vi "Rx_with scope_delta time.vi"() -> ()   [LabVIEW 2021]
uses:
  use with scope/states_for scope.ctl
  <instrlib>/niScope/Controls/niScope trigger source digital.ctl
  use with scope/scope trig type.ctl
  CTL/user config.ctl
  <vilib>/userdefined/High Color/nirio_resource_hc.ctl
  classes/5785_3.2GHz_one channel/5785_3.2GHz_one channel.lvclass
  C:/Users/PXIe8108_Demo/Documents/CHAIM DATA/chaim/5785_sync_for_elbit/tx_pulse/pulse Tx Folder_lv_21/EMEA_ADG_EW_Multi_Emitter_Scenarios/classes/device_type/device_type.lvclass
  classes/5785_2_x_1600MHz/5785_2_x_1600MHz.lvclass
  <instrlib>/niScope/Configure/Trigger/niScope Configure Trigger Edge.vi
  <instrlib>/niScope/Configure/Trigger/niScope Configure Trigger Digital.vi
  <instrlib>/niScope/Acquire/Fetch/niScope Multi Fetch WDT.vi
  <vilib>/Analysis/1siggen.llb/Ramp Pattern by Delta.vi
  classes/device_type/device_type.lvclass
  <vilib>/Analysis/NI_AALBase.lvlib
panel:
  in  "mode":T1(ring)=enum."5785 - 2*180MHz"
  in  "num of nano between channels":dbl
  out "delta range":cluster{dbl[], dbl[]}[](graph)=[{[200000.0, 200000.0, 200000.0, 200000.0, 200000.0, 200000.0, 200000.0, 200000.0, 200000.0, 200000.0, 200000.0, 200000.0, 200000.0, 200000.0, 200000.0, 200000.0, 200000.0, 200000.0, 200000.0, 200000.0, 200000.0, 200000.0, 200000.0, 200000.0, 200000.0, 200000.0, 200000.0, 200000.0, 200000.0, 200000.0, 200000.0, 200000.0, 200000.0, 200000.0, 200000.0, 200000.0, 200000.0, 200000.0, 200000.0, 200000.0, 200000.0, 200000.0, 200000.0, 200000.0, 200000.0, 200000.0, 200000.0, 200000.0, 200000.0, 200000.0, 200000.0, 200000.0, 200000.0, 200000.0, 200000.0, 200000.0, 200000.0, 200000.0, 200000.0, 200000.0, 200000.0, 200000.0, 200000.0, 200000.0, 200000.0, 200000.0, 200000.0, 200000.0, 200000.0, 200000.0, 200000.0, 200000.0, 200000.0, 200000.0, 200000.0, 200000.0, 200000.0, 200000.0, 200000.0, 200000.0, 200000.0, 200000.0, 200000.0, 200000.0, 200000.0, 200000.0, 200000.0, 200000.0, 200000.0, 200000.0, 200000.0, 200000.0, 200000.0, 200000.0, 200000.0, 200000.0, 200000.0, 200000.0, 200000.0, 200000.0, 200000.0, 200000.0, 200000.0, 200000.0, 200000.0, 200000.0, 200000.0, 200000.0, 200000.0, 200000.0, 200000.0, 200000.0, 200000.0, 200000.0, 200000.0, 200000.0, 200000.0, 200000.0, 200000.0, 200000.0, 200000.0, 200000.0, 200000.0, 200000.0, 200000.0, 200000.0, 200000.0, 200000.0, 200000.0, 200000.0, 200000.0, 200000.0, 200000.0, 200000.0, 200000.0, 200000.0, 200000.0, 200000.0, 200000.0, 200000.0, 200000.0, 200000.0, 200000.0, 200000.0, 200000.0, 200000.0, 200000.0, 200000.0, 200000.0, 200000.0, 200000.0, 200000.0, 200000.0, 200000.0, 200000.0, 200000.0, 200000.0, 200000.0, 200000.0, 200000.0, 200000.0, 200000.0], [-1.1815539075178094e-09, -1.1735940937302077e-09, 1.5173838718910703e-08, 1.1955568102002144e-08, 9.78047503704438e-09, 8.264037714514417e-09, 1.529550371572841e-08, 6.153523621009663e-09, 1.1997855926281773e-08, 1.0927362590376289e-08, 9.887324902811088e-09, 9.038956474978476e-09, 8.292742399894633e-09, 1.2053931898903102e-08, 1.538426720065763e-08, 6.832846135215369e-09, 1.3740200297546108e-08, 9.46442253064597e-09, -1.1883506176644005e-09, 2.0508825034904294e-08, 1.5174786625616252e-08, 1.1935071282531135e-08, 9.80493401925778e-09, 8.257336005754769e-09, 7.0956615944276564e-09, 1.3487845511222259e-08, 1.2094480889406986e-08, 1.089261531442171e-08, 9.913567475194577e-09, 1.910663676209515e-08, 1.3123609836224933e-08, 1.1936135569633917e-08, 7.184052554087248e-09, 6.482600684801582e-09, 9.916355201753322e-09, 9.171984461823013e-09, -1.1852903081453406e-09, 2.050388125119498e-08, 1.518068337268196e-08, 1.1954260133113712e-08, 2.0742580365296452e-08, 1.7653907625202556e-08, 1.5293914297246374e-08, 1.3515559364203364e-08, 1.8667553143179976e-08, 1.0837617655762007e-08, 9.826992215344217e-09, 9.018459328566678e-09, 8.301810464903247e-09, 1.2225356932776049e-08, 1.1088317456725054e-08, 1.429163756670896e-08, 6.338322277762927e-09, 5.658937157317996e-09, -1.1859513377188706e-09, -1.1768632264807821e-09, 1.5176432920689697e-08, 1.1960557492042426e-08, 9.826527517207432e-09, 8.233890970330685e-09, 7.106771544471849e-09, 2.0819609779305756e-08, 1.2022157269413583e-08, 1.0826222265674733e-08, 4.390260251308792e-09, 9.068177768285387e-09, 1.7713380407029765e-08, 1.2032988585217391e-08, 1.553451803342905e-08, 6.7977589478599845e-09, 1.3492854561959393e-08, 9.043047258420847e-09, -1.1866718047880568e-09, -1.168161773402244e-09, 1.516217105332762e-08, 1.1939343025384006e-08, 2.0737754271691665e-08, 8.226647777832114e-09, 2.3577958129288165e-08, 1.3539817026490345e-08, 1.2010466453281697e-08, 1.0798456547886599e-08, 9.887342741386966e-09, 9.049870830215513e-09, 1.7723341785010418e-08, 1.2062780513672624e-08, 7.134556607343257e-09, 1.8398769060708582e-08, 1.3532338226772846e-08, 9.478644459473435e-09, -1.1899547685286963e-09, 2.049997443513712e-08, -1.1591381137724966e-09, 2.5083063203259373e-08, 9.758059998776298e-09, 8.208837169304024e-09, 1.5304059904417955e-08, 1.3471675031236374e-08, 1.2010095862450544e-08, 4.8943541112937966e-09, 9.79197639725171e-09, 1.914853386823088e-08, 3.4211602777591907e-09, 1.2148997898632662e-08, 1.5279760670114775e-08, 1.0727430374035612e-08, 1.3727227776777e-08, 1.2907506954052951e-08, -1.191432826651726e-09, 2.0503596927179026e-08, 1.5179772480379325e-08, 1.193806957207853e-08, 2.074233382298844e-08, 8.258454856963362e-09, 1.5303464599850122e-08, 1.3454025143035688e-08, 1.8635701396665535e-08, 1.08096553556039e-08, 1.544961444224464e-08, 1.4091503172612283e-08, 1.2992782005574555e-08, 7.700502410845366e-09, 1.1210650748561603e-08, 6.467270610376727e-09, 1.3712995129253251e-08, 1.2856573502731045e-08, -1.181519340199884e-09, -1.1714998059673236e-09, -1.1691399245522917e-09, 1.1969364891957958e-08, 9.795761374232825e-09, 8.270884490117896e-09, 1.5300446236424615e-08, 1.3469071767153218e-08, 5.4664782162406484e-09, 1.081140604884131e-08, 9.877482435957063e-09, 1.4114352450484876e-08, 1.3036773227341474e-08, 1.658650060215732e-08, 1.1136174022918568e-08, 1.048507574532414e-08, 9.919178641459439e-09, 9.384021313837729e-09, -1.1804014970548452e-09, 2.0508209247060586e-08, 1.5182008155912626e-08, 1.1923188593576197e-08, 9.820071642228868e-09, 8.22439682368422e-09, 1.528007450030418e-08, 6.189352332078852e-09, 5.429137062910013e-09, 1.083287087896606e-08, 9.920461693149992e-09, 1.4080041759309825e-08, 1.3051713066059164e-08, 1.64067511016503e-08, 1.5338904302811716e-08, 1.4289069495361764e-08, 1.7299293319252322e-08, 9.347776307340245e-09]}, {[200000.0, 200000.0, 200000.0, 200000.0, 200000.0, 200000.0, 200000.0, 200000.0, 200000.0, 200000.0, 200000.0, 200000.0, 200000.0, 200000.0, 200000.0, 200000.0, 200000.0, 200000.0, 200000.0, 200000.0, 200000.0, 200000.0, 200000.0, 200000.0, 200000.0, 200000.0, 200000.0, 200000.0, 200000.0, 200000.0, 200000.0, 200000.0, 200000.0, 200000.0, 200000.0, 200000.0, 200000.0, 200000.0, 200000.0, 200000.0, 200000.0, 200000.0, 200000.0, 200000.0, 200000.0, 200000.0, 200000.0, 200000.0, 200000.0, 200000.0, 200000.0, 200000.0, 200000.0, 200000.0, 200000.0, 200000.0, 200000.0, 200000.0, 200000.0, 200000.0, 200000.0, 200000.0, 200000.0, 200000.0, 200000.0, 200000.0, 200000.0, 200000.0, 200000.0, 200000.0, 200000.0, 200000.0, 200000.0, 200000.0, 200000.0, 200000.0, 200000.0, 200000.0, 200000.0, 200000.0, 200000.0, 200000.0, 200000.0, 200000.0, 200000.0, 200000.0, 200000.0, 200000.0, 200000.0, 200000.0, 200000.0, 200000.0, 200000.0, 200000.0, 200000.0, 200000.0, 200000.0, 200000.0, 200000.0, 200000.0, 200000.0, 200000.0, 200000.0, 200000.0, 200000.0, 200000.0, 200000.0, 200000.0, 200000.0, 200000.0, 200000.0, 200000.0, 200000.0, 200000.0, 200000.0, 200000.0, 200000.0, 200000.0, 200000.0, 200000.0, 200000.0, 200000.0, 200000.0, 200000.0, 200000.0, 200000.0, 200000.0, 200000.0, 200000.0, 200000.0, 200000.0, 200000.0, 200000.0, 200000.0, 200000.0, 200000.0, 200000.0, 200000.0, 200000.0, 200000.0, 200000.0, 200000.0, 200000.0, 200000.0, 200000.0, 200000.0, 200000.0, 200000.0, 200000.0, 200000.0, 200000.0, 200000.0, 200000.0, 200000.0, 200000.0, 200000.0, 200000.0, 200000.0, 200000.0, 200000.0, 200000.0, 200000.0], [-5.2758537970250475e-09, -2.3407127689698245e-08, -6.722534446966602e-08, -5.429207686641021e-08, -1.265982775845332e-08, -6.769754615254933e-08, -1.6814595948671923e-09, -1.6661246864008718e-09, 2.6311391523241763e-07, 7.060455673366086e-08, -2.3770296792546288e-08, -8.333200363824145e-08, 5.990766722183907e-08, 1.6021572508569807e-08, 2.4549190990626813e-09, 2.5667595537542367e-08, -1.0133894762832206e-07, -4.364431243934669e-08, -2.6211028081248513e-09, -1.6764325760188514e-09, -1.4914255569522503e-07, -2.1211513884708985e-07, -1.1154114926223411e-07, 1.869374399444787e-07, -2.6460591026663317e-08, 2.771784418503521e-08, -2.201582827860373e-07, 4.046376852522371e-08, -2.668379908581963e-07, 3.422693380492274e-09, -1.7044445517705753e-09, -1.4839517075452024e-09, -9.715651885296684e-08, -1.4154818977462128e-09, -1.4033206062274986e-09, -1.4896887212409638e-09, -2.5997224274324252e-09, -1.6870750182657504e-09, -5.08418616282288e-08, -1.0689385669922922e-07, -3.463926962724654e-08, -1.0541058162089903e-07, 6.571010454441421e-09, 4.979177155462094e-08, 1.1563407812372316e-08, 1.187737823124975e-07, -1.5632612548315664e-07, -1.6481191426864826e-09, -8.695774586983025e-08, -1.5646854514456355e-07, -1.5836919521214442e-09, -9.151627552014543e-08, -2.375825364793418e-08, -1.4867069934960455e-09, 2.9570964601321612e-08, -1.68416051218519e-09, -1.327650510650943e-07, -6.74456698103575e-08, 1.3012938247543062e-07, -5.826020104213385e-08, -4.298418124335585e-08, -1.6306430794880725e-09, -1.65268333053682e-09, 4.34922378549818e-09, 1.8611463038435904e-07, -3.179790970514412e-07, 4.571838881932199e-08, -3.263085527048679e-08, -1.6103344403090887e-09, -5.2450860559660945e-08, -6.069644739819924e-08, -9.960683704963886e-08, -2.7812305574072528e-09, -2.3407655791426077e-08, -1.680400427884888e-09, 1.2983798663063207e-07, -1.2250856097332436e-07, -1.9028673857010436e-07, -6.776840066893492e-08, 1.526710163182812e-07, -1.4069603167161114e-07, -1.3729507627873682e-08, -1.2322045791811543e-07, -1.5640510332770646e-09, -1.114380489231553e-08, 4.6973823060106954e-08, -2.2434419115853962e-08, -1.7172170262900182e-09, -1.4922106679473074e-07, -1.375437327986583e-09, -3.3200913137756288e-09, -8.858227864420042e-08, 1.4700512176577468e-08, -1.6891061169211753e-09, -7.857818397136871e-08, -6.76943390746601e-08, 3.137742357105017e-08, 5.6726777313277125e-09, -1.4913748137338554e-08, -2.5779230802343227e-08, -1.1766951875201194e-07, -8.330288391152863e-08, -1.110966835586587e-08, -2.670595320973196e-07, -1.7175967923381833e-07, 5.692949443269754e-08, -1.6040403344319202e-09, -1.1010502003676957e-07, -2.5993297878187153e-09, -1.6872152113122865e-09, -1.6665501618990676e-09, -2.7985244101309217e-08, 9.298273379483727e-09, 7.726421110320371e-09, 3.9630540137866045e-08, -2.3692681606730914e-07, 1.8177111647382845e-08, 1.6381107255979442e-08, 6.45988679313101e-08, -6.797660859823227e-08, 1.1204547074270668e-07, 8.679257690348895e-08, 6.055344777908176e-08, -2.117703055985039e-08, 7.578887686054223e-08, -8.63803369246889e-09, -2.601511100458447e-09, -1.6848717768210918e-09, -8.361155117555755e-08, 3.777623066526139e-08, -1.66458464711532e-07, -1.1109763558150735e-08, -7.602773881788599e-08, 2.6294636838844747e-07, -8.776025092410856e-08, -6.79101360932109e-08, -2.928374278978445e-08, 2.738065298111877e-07, -2.338121665910352e-07, -1.6695078473887406e-09, -8.461940371126403e-08, 2.24946505028056e-09, -3.1187497843243186e-08, 1.5777326026628725e-08, -2.6682210018159824e-09, 2.0040185065031982e-08, -1.6872021939605476e-09, -1.6708021246129648e-09, 2.0281507924827746e-08, -1.6701500906609e-09, 5.615237306245836e-08, -4.5785180069925264e-08, -1.6699399421107956e-09, -1.974793375823647e-08, 2.8002474203405436e-07, -1.5979692357477035e-07, -1.6879449682077394e-09, 2.9279428828228268e-08, -1.6210599262383766e-09, -1.3368764323415235e-08, 2.779946841171477e-08, -8.912615016765195e-08]}, {[200000.0, 200000.0, 200000.0, 200000.0, 200000.0, 200000.0, 200000.0, 200000.0, 200000.0, 200000.0, 200000.0, 200000.0, 200000.0, 200000.0, 200000.0, 200000.0, 200000.0, 200000.0, 200000.0, 200000.0, 200000.0, 200000.0, 200000.0, 200000.0, 200000.0, 200000.0, 200000.0, 200000.0, 200000.0, 200000.0, 200000.0, 200000.0, 200000.0, 200000.0, 200000.0, 200000.0, 200000.0, 200000.0, 200000.0, 200000.0, 200000.0, 200000.0, 200000.0, 200000.0, 200000.0, 200000.0, 200000.0, 200000.0, 200000.0, 200000.0, 200000.0, 200000.0, 200000.0, 200000.0, 200000.0, 200000.0, 200000.0, 200000.0, 200000.0, 200000.0, 200000.0, 200000.0, 200000.0, 200000.0, 200000.0, 200000.0, 200000.0, 200000.0, 200000.0, 200000.0, 200000.0, 200000.0, 200000.0, 200000.0, 200000.0, 200000.0, 200000.0, 200000.0, 200000.0, 200000.0, 200000.0, 200000.0, 200000.0, 200000.0, 200000.0, 200000.0, 200000.0, 200000.0, 200000.0, 200000.0, 200000.0, 200000.0, 200000.0, 200000.0, 200000.0, 200000.0, 200000.0, 200000.0, 200000.0, 200000.0, 200000.0, 200000.0, 200000.0, 200000.0, 200000.0, 200000.0, 200000.0, 200000.0, 200000.0, 200000.0, 200000.0, 200000.0, 200000.0, 200000.0, 200000.0, 200000.0, 200000.0, 200000.0, 200000.0, 200000.0, 200000.0, 200000.0, 200000.0, 200000.0, 200000.0, 200000.0, 200000.0, 200000.0, 200000.0, 200000.0, 200000.0, 200000.0, 200000.0, 200000.0, 200000.0, 200000.0, 200000.0, 200000.0, 200000.0, 200000.0, 200000.0, 200000.0, 200000.0, 200000.0, 200000.0, 200000.0, 200000.0, 200000.0, 200000.0, 200000.0, 200000.0, 200000.0, 200000.0, 200000.0, 200000.0, 200000.0, 200000.0, 200000.0, 200000.0, 200000.0, 200000.0, 200000.0], [-1.7749814823269846e-09, 1.7916497242287734e-09, 1.810030858742539e-09, 1.7622843523742631e-09, 1.790128987596836e-09, -7.591239673167002e-09, -6.438507502002176e-09, -5.514481092884671e-09, 1.7846586266532541e-09, -4.11769536313368e-09, 1.7282367827021517e-09, 1.8549817233579233e-09, 6.637878210714553e-09, 1.9506171769846697e-08, 1.7450234520831147e-09, -2.104156445490662e-09, -1.7553881366387942e-09, 1.7225313605740668e-09, 8.55821915762499e-10, 1.7910540758515708e-09, -1.1289434410749237e-07, 1.5961078651172575e-07, 1.2752211420226378e-08, 1.7156020832882496e-07, -2.790998933401192e-07, 1.795106326416135e-09, -1.7697934423995902e-07, 1.830049466143828e-09, 7.3156441754661505e-09, -8.370264219632372e-09, 1.892111062211916e-09, 1.9237002010457217e-09, -1.9692398519488053e-09, -1.7853011123952456e-09, -1.379460162506439e-09, 1.934421759969555e-08, 8.81783880002331e-10, 1.8057898015482352e-09, 1.7897386681521312e-09, 1.8122219059965573e-09, -9.191244989994448e-09, 1.8352211295976305e-09, 1.7543499617720956e-09, 1.7397789353155531e-09, 1.8411824457463809e-09, -4.245045999751892e-09, -1.8046205354604172e-07, 1.7591319564031438e-09, -1.2417493940913119e-08, -1.6191040982939304e-07, -2.2869246410555207e-09, 1.6727303515421227e-09, -5.517827092541847e-09, 5.141949368198402e-09, 8.293245125212707e-10, 1.7919849544530734e-09, 1.8109318249393255e-09, 1.767806403944269e-09, 1.9952939063706436e-07, 1.8045291647780688e-09, 1.8135523594217377e-09, 9.132958083134144e-09, -4.756782229524106e-09, 1.7780634230468423e-09, 7.3099776151590055e-09, 6.816042163118255e-09, 1.1240640289220027e-08, 1.6734723222325557e-09, 3.130030399346142e-07, -2.0910783499712125e-09, -1.9921912132995202e-09, -5.12793291854905e-09, 7.013775807106868e-10, 1.7959166439133696e-09, 1.8059124657069333e-09, 1.493616162445396e-08, 1.7824652628740297e-09, 2.0647735671186822e-08, 1.8131193301407621e-09, 1.5618133324038936e-07, 1.7874781763646753e-09, 1.8175690842675977e-09, -1.5285434376745253e-07, 1.8327746704919264e-09, -7.589546780346427e-09, 6.262374498764984e-09, -2.1930375333642586e-09, 5.7738439642009325e-09, 1.7687889691442252e-09, 5.247123713733163e-09, 1.6380919446237387e-10, 1.7924074603244662e-09, 1.8166623340803199e-09, 1.7901294152834453e-09, -9.161749687616248e-09, -7.625480377313215e-09, -6.46756274154177e-09, 9.139076100615784e-09, 1.8232319623581134e-09, 1.7103415188845247e-09, -9.226441835064907e-09, 1.742226669145748e-09, 6.580859854549635e-09, -2.590121800720226e-09, 1.0134401007124689e-08, 1.6586110266391188e-09, 5.35790876528481e-09, -9.96144644873566e-08, 8.858655306044967e-10, 1.810248641401995e-09, 1.8204800266772509e-09, 1.827525897405576e-09, -9.157252589869314e-09, -7.601911332714372e-09, 1.8169124716543593e-09, 1.7858749113045634e-09, 8.385745622077957e-09, -4.174609289679211e-09, 7.311240029521287e-09, -3.1910439292434603e-09, 1.7306726491427981e-09, 1.797852179442998e-09, 1.0139323838144774e-07, -2.1244258358725345e-09, 2.3907385512522888e-08, 1.6123738369555213e-09, 8.85242059128359e-10, 1.8070682415389456e-09, 1.7765487509546802e-09, 1.8111083562602289e-09, 1.81600947114639e-09, 1.7794284046278336e-09, 1.8337304288172164e-09, 1.8479100456344895e-09, -2.4314560706031044e-07, 1.7774576973635703e-09, 1.7314097517170012e-09, 1.9052965071884682e-07, -2.733420779486187e-09, -2.4605247770552526e-09, -2.369954527623486e-09, 1.7807079949066976e-09, -2.030338526959531e-09, 8.65108720465796e-09, 8.168054007808678e-10, 1.8061025098199025e-09, 1.816646474832669e-09, 1.8131524985074066e-09, 1.2799038003920578e-08, 1.8052098663290964e-09, 1.0090849893772975e-08, -5.5400895392871466e-09, -4.8145288588013506e-09, -1.0188812083390077e-08, 1.8360702333389783e-09, 1.7130488279159182e-09, 1.8827813584241087e-09, 1.6259373551001773e-09, 9.720785760920263e-08, 1.4690440165111795e-09, 1.489713418064639e-09, 5.059258201089688e-09]}]
  out "delta time (sec)":cluster{dbl[], dbl[]}[](graph)=[{[200000.0, 200000.0, 200000.0, 200000.0, 200000.0, 200000.0, 200000.0, 200000.0, 200000.0, 200000.0, 200000.0, 200000.0, 200000.0, 200000.0, 200000.0, 200000.0, 200000.0, 200000.0, 200000.0, 200000.0, 200000.0, 200000.0, 200000.0, 200000.0, 200000.0, 200000.0, 200000.0, 200000.0, 200000.0, 200000.0, 200000.0, 200000.0, 200000.0, 200000.0, 200000.0, 200000.0, 200000.0, 200000.0, 200000.0, 200000.0, 200000.0, 200000.0, 200000.0, 200000.0, 200000.0, 200000.0, 200000.0, 200000.0, 200000.0, 200000.0, 200000.0, 200000.0, 200000.0, 200000.0, 200000.0, 200000.0, 200000.0, 200000.0, 200000.0, 200000.0, 200000.0, 200000.0, 200000.0, 200000.0, 200000.0, 200000.0, 200000.0, 200000.0, 200000.0, 200000.0, 200000.0, 200000.0, 200000.0, 200000.0, 200000.0, 200000.0, 200000.0, 200000.0, 200000.0, 200000.0, 200000.0, 200000.0, 200000.0, 200000.0, 200000.0, 200000.0, 200000.0, 200000.0, 200000.0, 200000.0, 200000.0, 200000.0, 200000.0, 200000.0, 200000.0, 200000.0, 200000.0, 200000.0, 200000.0, 200000.0, 200000.0, 200000.0, 200000.0, 200000.0, 200000.0, 200000.0, 200000.0, 200000.0, 200000.0, 200000.0, 200000.0, 200000.0, 200000.0, 200000.0, 200000.0, 200000.0, 200000.0, 200000.0, 200000.0, 200000.0, 200000.0, 200000.0, 200000.0, 200000.0, 200000.0, 200000.0, 200000.0, 200000.0, 200000.0, 200000.0, 200000.0, 200000.0, 200000.0, 200000.0, 200000.0, 200000.0, 200000.0, 200000.0, 200000.0, 200000.0, 200000.0, 200000.0, 200000.0, 200000.0, 200000.0, 200000.0, 200000.0, 200000.0, 200000.0, 200000.0, 200000.0, 200000.0, 200000.0, 200000.0, 200000.0, 200000.0, 200000.0, 200000.0, 200000.0, 200000.0, 200000.0, 200000.0], [-1.1815539075178094e-09, -1.1735940937302077e-09, 1.5173838718910703e-08, 1.1955568102002144e-08, 9.78047503704438e-09, 8.264037714514417e-09, 1.529550371572841e-08, 6.153523621009663e-09, 1.1997855926281773e-08, 1.0927362590376289e-08, 9.887324902811088e-09, 9.038956474978476e-09, 8.292742399894633e-09, 1.2053931898903102e-08, 1.538426720065763e-08, 6.832846135215369e-09, 1.3740200297546108e-08, 9.46442253064597e-09, -1.1883506176644005e-09, 2.0508825034904294e-08, 1.5174786625616252e-08, 1.1935071282531135e-08, 9.80493401925778e-09, 8.257336005754769e-09, 7.0956615944276564e-09, 1.3487845511222259e-08, 1.2094480889406986e-08, 1.089261531442171e-08, 9.913567475194577e-09, 1.910663676209515e-08, 1.3123609836224933e-08, 1.1936135569633917e-08, 7.184052554087248e-09, 6.482600684801582e-09, 9.916355201753322e-09, 9.171984461823013e-09, -1.1852903081453406e-09, 2.050388125119498e-08, 1.518068337268196e-08, 1.1954260133113712e-08, 2.0742580365296452e-08, 1.7653907625202556e-08, 1.5293914297246374e-08, 1.3515559364203364e-08, 1.8667553143179976e-08, 1.0837617655762007e-08, 9.826992215344217e-09, 9.018459328566678e-09, 8.301810464903247e-09, 1.2225356932776049e-08, 1.1088317456725054e-08, 1.429163756670896e-08, 6.338322277762927e-09, 5.658937157317996e-09, -1.1859513377188706e-09, -1.1768632264807821e-09, 1.5176432920689697e-08, 1.1960557492042426e-08, 9.826527517207432e-09, 8.233890970330685e-09, 7.106771544471849e-09, 2.0819609779305756e-08, 1.2022157269413583e-08, 1.0826222265674733e-08, 4.390260251308792e-09, 9.068177768285387e-09, 1.7713380407029765e-08, 1.2032988585217391e-08, 1.553451803342905e-08, 6.7977589478599845e-09, 1.3492854561959393e-08, 9.043047258420847e-09, -1.1866718047880568e-09, -1.168161773402244e-09, 1.516217105332762e-08, 1.1939343025384006e-08, 2.0737754271691665e-08, 8.226647777832114e-09, 2.3577958129288165e-08, 1.3539817026490345e-08, 1.2010466453281697e-08, 1.0798456547886599e-08, 9.887342741386966e-09, 9.049870830215513e-09, 1.7723341785010418e-08, 1.2062780513672624e-08, 7.134556607343257e-09, 1.8398769060708582e-08, 1.3532338226772846e-08, 9.478644459473435e-09, -1.1899547685286963e-09, 2.049997443513712e-08, -1.1591381137724966e-09, 2.5083063203259373e-08, 9.758059998776298e-09, 8.208837169304024e-09, 1.5304059904417955e-08, 1.3471675031236374e-08, 1.2010095862450544e-08, 4.8943541112937966e-09, 9.79197639725171e-09, 1.914853386823088e-08, 3.4211602777591907e-09, 1.2148997898632662e-08, 1.5279760670114775e-08, 1.0727430374035612e-08, 1.3727227776777e-08, 1.2907506954052951e-08, -1.191432826651726e-09, 2.0503596927179026e-08, 1.5179772480379325e-08, 1.193806957207853e-08, 2.074233382298844e-08, 8.258454856963362e-09, 1.5303464599850122e-08, 1.3454025143035688e-08, 1.8635701396665535e-08, 1.08096553556039e-08, 1.544961444224464e-08, 1.4091503172612283e-08, 1.2992782005574555e-08, 7.700502410845366e-09, 1.1210650748561603e-08, 6.467270610376727e-09, 1.3712995129253251e-08, 1.2856573502731045e-08, -1.181519340199884e-09, -1.1714998059673236e-09, -1.1691399245522917e-09, 1.1969364891957958e-08, 9.795761374232825e-09, 8.270884490117896e-09, 1.5300446236424615e-08, 1.3469071767153218e-08, 5.4664782162406484e-09, 1.081140604884131e-08, 9.877482435957063e-09, 1.4114352450484876e-08, 1.3036773227341474e-08, 1.658650060215732e-08, 1.1136174022918568e-08, 1.048507574532414e-08, 9.919178641459439e-09, 9.384021313837729e-09, -1.1804014970548452e-09, 2.0508209247060586e-08, 1.5182008155912626e-08, 1.1923188593576197e-08, 9.820071642228868e-09, 8.22439682368422e-09, 1.528007450030418e-08, 6.189352332078852e-09, 5.429137062910013e-09, 1.083287087896606e-08, 9.920461693149992e-09, 1.4080041759309825e-08, 1.3051713066059164e-08, 1.64067511016503e-08, 1.5338904302811716e-08, 1.4289069495361764e-08, 1.7299293319252322e-08, 9.347776307340245e-09]}, {[200000.0, 200000.0, 200000.0, 200000.0, 200000.0, 200000.0, 200000.0, 200000.0, 200000.0, 200000.0, 200000.0, 200000.0, 200000.0, 200000.0, 200000.0, 200000.0, 200000.0, 200000.0, 200000.0, 200000.0, 200000.0, 200000.0, 200000.0, 200000.0, 200000.0, 200000.0, 200000.0, 200000.0, 200000.0, 200000.0, 200000.0, 200000.0, 200000.0, 200000.0, 200000.0, 200000.0, 200000.0, 200000.0, 200000.0, 200000.0, 200000.0, 200000.0, 200000.0, 200000.0, 200000.0, 200000.0, 200000.0, 200000.0, 200000.0, 200000.0, 200000.0, 200000.0, 200000.0, 200000.0, 200000.0, 200000.0, 200000.0, 200000.0, 200000.0, 200000.0, 200000.0, 200000.0, 200000.0, 200000.0, 200000.0, 200000.0, 200000.0, 200000.0, 200000.0, 200000.0, 200000.0, 200000.0, 200000.0, 200000.0, 200000.0, 200000.0, 200000.0, 200000.0, 200000.0, 200000.0, 200000.0, 200000.0, 200000.0, 200000.0, 200000.0, 200000.0, 200000.0, 200000.0, 200000.0, 200000.0, 200000.0, 200000.0, 200000.0, 200000.0, 200000.0, 200000.0, 200000.0, 200000.0, 200000.0, 200000.0, 200000.0, 200000.0, 200000.0, 200000.0, 200000.0, 200000.0, 200000.0, 200000.0, 200000.0, 200000.0, 200000.0, 200000.0, 200000.0, 200000.0, 200000.0, 200000.0, 200000.0, 200000.0, 200000.0, 200000.0, 200000.0, 200000.0, 200000.0, 200000.0, 200000.0, 200000.0, 200000.0, 200000.0, 200000.0, 200000.0, 200000.0, 200000.0, 200000.0, 200000.0, 200000.0, 200000.0, 200000.0, 200000.0, 200000.0, 200000.0, 200000.0, 200000.0, 200000.0, 200000.0, 200000.0, 200000.0, 200000.0, 200000.0, 200000.0, 200000.0, 200000.0, 200000.0, 200000.0, 200000.0, 200000.0, 200000.0, 200000.0, 200000.0, 200000.0, 200000.0, 200000.0, 200000.0], [-5.2758537970250475e-09, -2.3407127689698245e-08, -6.722534446966602e-08, -5.429207686641021e-08, -1.265982775845332e-08, -6.769754615254933e-08, -1.6814595948671923e-09, -1.6661246864008718e-09, 2.6311391523241763e-07, 7.060455673366086e-08, -2.3770296792546288e-08, -8.333200363824145e-08, 5.990766722183907e-08, 1.6021572508569807e-08, 2.4549190990626813e-09, 2.5667595537542367e-08, -1.0133894762832206e-07, -4.364431243934669e-08, -2.6211028081248513e-09, -1.6764325760188514e-09, -1.4914255569522503e-07, -2.1211513884708985e-07, -1.1154114926223411e-07, 1.869374399444787e-07, -2.6460591026663317e-08, 2.771784418503521e-08, -2.201582827860373e-07, 4.046376852522371e-08, -2.668379908581963e-07, 3.422693380492274e-09, -1.7044445517705753e-09, -1.4839517075452024e-09, -9.715651885296684e-08, -1.4154818977462128e-09, -1.4033206062274986e-09, -1.4896887212409638e-09, -2.5997224274324252e-09, -1.6870750182657504e-09, -5.08418616282288e-08, -1.0689385669922922e-07, -3.463926962724654e-08, -1.0541058162089903e-07, 6.571010454441421e-09, 4.979177155462094e-08, 1.1563407812372316e-08, 1.187737823124975e-07, -1.5632612548315664e-07, -1.6481191426864826e-09, -8.695774586983025e-08, -1.5646854514456355e-07, -1.5836919521214442e-09, -9.151627552014543e-08, -2.375825364793418e-08, -1.4867069934960455e-09, 2.9570964601321612e-08, -1.68416051218519e-09, -1.327650510650943e-07, -6.74456698103575e-08, 1.3012938247543062e-07, -5.826020104213385e-08, -4.298418124335585e-08, -1.6306430794880725e-09, -1.65268333053682e-09, 4.34922378549818e-09, 1.8611463038435904e-07, -3.179790970514412e-07, 4.571838881932199e-08, -3.263085527048679e-08, -1.6103344403090887e-09, -5.2450860559660945e-08, -6.069644739819924e-08, -9.960683704963886e-08, -2.7812305574072528e-09, -2.3407655791426077e-08, -1.680400427884888e-09, 1.2983798663063207e-07, -1.2250856097332436e-07, -1.9028673857010436e-07, -6.776840066893492e-08, 1.526710163182812e-07, -1.4069603167161114e-07, -1.3729507627873682e-08, -1.2322045791811543e-07, -1.5640510332770646e-09, -1.114380489231553e-08, 4.6973823060106954e-08, -2.2434419115853962e-08, -1.7172170262900182e-09, -1.4922106679473074e-07, -1.375437327986583e-09, -3.3200913137756288e-09, -8.858227864420042e-08, 1.4700512176577468e-08, -1.6891061169211753e-09, -7.857818397136871e-08, -6.76943390746601e-08, 3.137742357105017e-08, 5.6726777313277125e-09, -1.4913748137338554e-08, -2.5779230802343227e-08, -1.1766951875201194e-07, -8.330288391152863e-08, -1.110966835586587e-08, -2.670595320973196e-07, -1.7175967923381833e-07, 5.692949443269754e-08, -1.6040403344319202e-09, -1.1010502003676957e-07, -2.5993297878187153e-09, -1.6872152113122865e-09, -1.6665501618990676e-09, -2.7985244101309217e-08, 9.298273379483727e-09, 7.726421110320371e-09, 3.9630540137866045e-08, -2.3692681606730914e-07, 1.8177111647382845e-08, 1.6381107255979442e-08, 6.45988679313101e-08, -6.797660859823227e-08, 1.1204547074270668e-07, 8.679257690348895e-08, 6.055344777908176e-08, -2.117703055985039e-08, 7.578887686054223e-08, -8.63803369246889e-09, -2.601511100458447e-09, -1.6848717768210918e-09, -8.361155117555755e-08, 3.777623066526139e-08, -1.66458464711532e-07, -1.1109763558150735e-08, -7.602773881788599e-08, 2.6294636838844747e-07, -8.776025092410856e-08, -6.79101360932109e-08, -2.928374278978445e-08, 2.738065298111877e-07, -2.338121665910352e-07, -1.6695078473887406e-09, -8.461940371126403e-08, 2.24946505028056e-09, -3.1187497843243186e-08, 1.5777326026628725e-08, -2.6682210018159824e-09, 2.0040185065031982e-08, -1.6872021939605476e-09, -1.6708021246129648e-09, 2.0281507924827746e-08, -1.6701500906609e-09, 5.615237306245836e-08, -4.5785180069925264e-08, -1.6699399421107956e-09, -1.974793375823647e-08, 2.8002474203405436e-07, -1.5979692357477035e-07, -1.6879449682077394e-09, 2.9279428828228268e-08, -1.6210599262383766e-09, -1.3368764323415235e-08, 2.779946841171477e-08, -8.912615016765195e-08]}, {[200000.0, 200000.0, 200000.0, 200000.0, 200000.0, 200000.0, 200000.0, 200000.0, 200000.0, 200000.0, 200000.0, 200000.0, 200000.0, 200000.0, 200000.0, 200000.0, 200000.0, 200000.0, 200000.0, 200000.0, 200000.0, 200000.0, 200000.0, 200000.0, 200000.0, 200000.0, 200000.0, 200000.0, 200000.0, 200000.0, 200000.0, 200000.0, 200000.0, 200000.0, 200000.0, 200000.0, 200000.0, 200000.0, 200000.0, 200000.0, 200000.0, 200000.0, 200000.0, 200000.0, 200000.0, 200000.0, 200000.0, 200000.0, 200000.0, 200000.0, 200000.0, 200000.0, 200000.0, 200000.0, 200000.0, 200000.0, 200000.0, 200000.0, 200000.0, 200000.0, 200000.0, 200000.0, 200000.0, 200000.0, 200000.0, 200000.0, 200000.0, 200000.0, 200000.0, 200000.0, 200000.0, 200000.0, 200000.0, 200000.0, 200000.0, 200000.0, 200000.0, 200000.0, 200000.0, 200000.0, 200000.0, 200000.0, 200000.0, 200000.0, 200000.0, 200000.0, 200000.0, 200000.0, 200000.0, 200000.0, 200000.0, 200000.0, 200000.0, 200000.0, 200000.0, 200000.0, 200000.0, 200000.0, 200000.0, 200000.0, 200000.0, 200000.0, 200000.0, 200000.0, 200000.0, 200000.0, 200000.0, 200000.0, 200000.0, 200000.0, 200000.0, 200000.0, 200000.0, 200000.0, 200000.0, 200000.0, 200000.0, 200000.0, 200000.0, 200000.0, 200000.0, 200000.0, 200000.0, 200000.0, 200000.0, 200000.0, 200000.0, 200000.0, 200000.0, 200000.0, 200000.0, 200000.0, 200000.0, 200000.0, 200000.0, 200000.0, 200000.0, 200000.0, 200000.0, 200000.0, 200000.0, 200000.0, 200000.0, 200000.0, 200000.0, 200000.0, 200000.0, 200000.0, 200000.0, 200000.0, 200000.0, 200000.0, 200000.0, 200000.0, 200000.0, 200000.0, 200000.0, 200000.0, 200000.0, 200000.0, 200000.0, 200000.0], [-1.7749814823269846e-09, 1.7916497242287734e-09, 1.810030858742539e-09, 1.7622843523742631e-09, 1.790128987596836e-09, -7.591239673167002e-09, -6.438507502002176e-09, -5.514481092884671e-09, 1.7846586266532541e-09, -4.11769536313368e-09, 1.7282367827021517e-09, 1.8549817233579233e-09, 6.637878210714553e-09, 1.9506171769846697e-08, 1.7450234520831147e-09, -2.104156445490662e-09, -1.7553881366387942e-09, 1.7225313605740668e-09, 8.55821915762499e-10, 1.7910540758515708e-09, -1.1289434410749237e-07, 1.5961078651172575e-07, 1.2752211420226378e-08, 1.7156020832882496e-07, -2.790998933401192e-07, 1.795106326416135e-09, -1.7697934423995902e-07, 1.830049466143828e-09, 7.3156441754661505e-09, -8.370264219632372e-09, 1.892111062211916e-09, 1.9237002010457217e-09, -1.9692398519488053e-09, -1.7853011123952456e-09, -1.379460162506439e-09, 1.934421759969555e-08, 8.81783880002331e-10, 1.8057898015482352e-09, 1.7897386681521312e-09, 1.8122219059965573e-09, -9.191244989994448e-09, 1.8352211295976305e-09, 1.7543499617720956e-09, 1.7397789353155531e-09, 1.8411824457463809e-09, -4.245045999751892e-09, -1.8046205354604172e-07, 1.7591319564031438e-09, -1.2417493940913119e-08, -1.6191040982939304e-07, -2.2869246410555207e-09, 1.6727303515421227e-09, -5.517827092541847e-09, 5.141949368198402e-09, 8.293245125212707e-10, 1.7919849544530734e-09, 1.8109318249393255e-09, 1.767806403944269e-09, 1.9952939063706436e-07, 1.8045291647780688e-09, 1.8135523594217377e-09, 9.132958083134144e-09, -4.756782229524106e-09, 1.7780634230468423e-09, 7.3099776151590055e-09, 6.816042163118255e-09, 1.1240640289220027e-08, 1.6734723222325557e-09, 3.130030399346142e-07, -2.0910783499712125e-09, -1.9921912132995202e-09, -5.12793291854905e-09, 7.013775807106868e-10, 1.7959166439133696e-09, 1.8059124657069333e-09, 1.493616162445396e-08, 1.7824652628740297e-09, 2.0647735671186822e-08, 1.8131193301407621e-09, 1.5618133324038936e-07, 1.7874781763646753e-09, 1.8175690842675977e-09, -1.5285434376745253e-07, 1.8327746704919264e-09, -7.589546780346427e-09, 6.262374498764984e-09, -2.1930375333642586e-09, 5.7738439642009325e-09, 1.7687889691442252e-09, 5.247123713733163e-09, 1.6380919446237387e-10, 1.7924074603244662e-09, 1.8166623340803199e-09, 1.7901294152834453e-09, -9.161749687616248e-09, -7.625480377313215e-09, -6.46756274154177e-09, 9.139076100615784e-09, 1.8232319623581134e-09, 1.7103415188845247e-09, -9.226441835064907e-09, 1.742226669145748e-09, 6.580859854549635e-09, -2.590121800720226e-09, 1.0134401007124689e-08, 1.6586110266391188e-09, 5.35790876528481e-09, -9.96144644873566e-08, 8.858655306044967e-10, 1.810248641401995e-09, 1.8204800266772509e-09, 1.827525897405576e-09, -9.157252589869314e-09, -7.601911332714372e-09, 1.8169124716543593e-09, 1.7858749113045634e-09, 8.385745622077957e-09, -4.174609289679211e-09, 7.311240029521287e-09, -3.1910439292434603e-09, 1.7306726491427981e-09, 1.797852179442998e-09, 1.0139323838144774e-07, -2.1244258358725345e-09, 2.3907385512522888e-08, 1.6123738369555213e-09, 8.85242059128359e-10, 1.8070682415389456e-09, 1.7765487509546802e-09, 1.8111083562602289e-09, 1.81600947114639e-09, 1.7794284046278336e-09, 1.8337304288172164e-09, 1.8479100456344895e-09, -2.4314560706031044e-07, 1.7774576973635703e-09, 1.7314097517170012e-09, 1.9052965071884682e-07, -2.733420779486187e-09, -2.4605247770552526e-09, -2.369954527623486e-09, 1.7807079949066976e-09, -2.030338526959531e-09, 8.65108720465796e-09, 8.168054007808678e-10, 1.8061025098199025e-09, 1.816646474832669e-09, 1.8131524985074066e-09, 1.2799038003920578e-08, 1.8052098663290964e-09, 1.0090849893772975e-08, -5.5400895392871466e-09, -4.8145288588013506e-09, -1.0188812083390077e-08, 1.8360702333389783e-09, 1.7130488279159182e-09, 1.8827813584241087e-09, 1.6259373551001773e-09, 9.720785760920263e-08, 1.4690440165111795e-09, 1.489713418064639e-09, 5.059258201089688e-09]}]
  in  "niqiest band":dbl[](array[numeric])=[0.0]
  in  "clear":bool=TRUE
  out "saturate":bool
  in  "atenuattion (dB)":dbl format="%#_13g"
  in  "Min. Sample Rate":dbl=1250000000.0 format="%#.3p"
  in  "maximum input frequency":dbl=800000000.0 format="%#_13p"
  in  "input impedance":u32(ring)=2 items=["1 mega ohm"=0, "50 ohms"=2]
  in  "keep data":bool=TRUE
  in  "test mode":bool=TRUE
  in  "save file":bool=TRUE
  in  "file path":path=path "C:/Users/PXIe8108_Demo/Documents/CHAIM DATA/chaim/5785_sync_for_elbit/tx_pulse/pulse Tx Folder_lv_21/EMEA_ADG_EW_Multi_Emitter_Scenarios/data/scope_cal_file.tdms"
  in  "num of recordes":dbl=1.0 format="%#_13g"
  in  "num of devices":dbl=2.0 format="%#_13g"
  in  "gen PDW file":bool
  in  "frequncy comb":cluster{"start":dbl, "end":dbl, "delta":dbl}={"start"=20000000.0, "end"=300000000.0, "delta"=15000000.0} {"delta" format="%#_6p"; "end" format="%#_6p"; "start" format="%#_6p"}
  out "spectrum":cluster{"f0":dbl, "df":dbl, "magnitude":dbl[]}[](graph)=[{"f0"=-625000000.0, "df"=10000.0, "magnitude"=array[125000 elements]}, {"f0"=-625000000.0, "df"=10000.0, "magnitude"=array[125000 elements]}, {"f0"=-625000000.0, "df"=10000.0, "magnitude"=array[125000 elements]}, {"f0"=-625000000.0, "df"=10000.0, "magnitude"=array[125000 elements]}]
  in  "reset data":bool=TRUE
  in  "loop mode":bool=TRUE
  out "state":T2
  in  "cal":bool
  in  "Channel Name":string="0,1"
  in  "Resource Name":refnum<k15>="PXI1Slot6" caption="Resource Name(s)"
  in  "amplitude (dB)":dbl=-30.0 format="%#_13g"
  in  "record duration (s)":dbl=5e-05 format="%#_13p"
  out "scope":waveform(dbl)[](graph)=[{"t0"=timestamp(3784798982.6075587 s since 1904-01-01), "dt"=8e-10, "Y"=array[125000 elements]}, {"t0"=timestamp(3784798982.6075587 s since 1904-01-01), "dt"=8e-10, "Y"=array[125000 elements]}, {"t0"=timestamp(3784798982.6075587 s since 1904-01-01), "dt"=8e-10, "Y"=array[125000 elements]}, {"t0"=timestamp(3784798982.6075587 s since 1904-01-01), "dt"=8e-10, "Y"=array[125000 elements]}]
  # "scope delta time detection"
  # "RF setup"
  # "HW setup"
  # "Rx Data"
  # "scope mapping:\nchannel 0 => 5785_02 _0 \nchannel 1 => 5785_01 _0 \nchannel 2 => 5785_01 _1 \nchannel 3 => 5785_00 _1"
  # "SW setup"
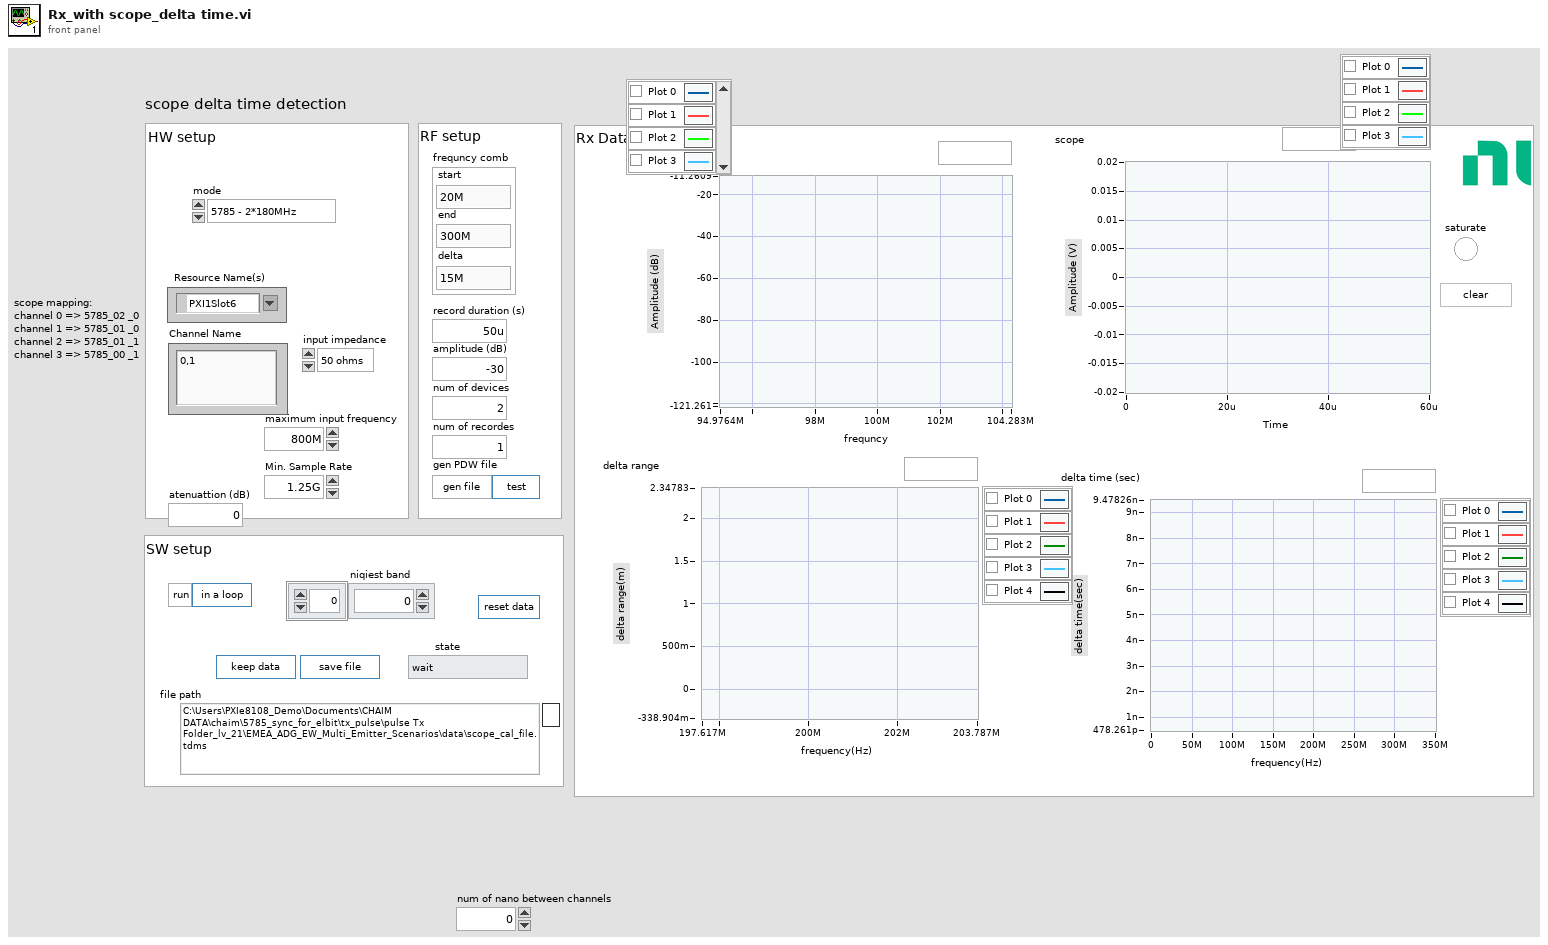
[diagram p1: front panel]
types:
  T1 = enum16{"USRP - 180MHz", "5785 - 2*180MHz", "5785 - 3.2GHz", "P2P - VST"}
  T2 = typedef "states_for scope.ctl" = enum16{"wait", "update ME config", "gen secenario", "INI ME", "INI scope", "trig", "close ME", "run mesearment", "save cal data", "get file data", "gen PDW file", "keep the data", "reset memory data", "prime the fifo"}
  T3 = typedef "niScope trigger source digital.ctl" = string
  T4 = typedef "scope trig type.ctl" = enum16{"digital", "analog"}
  T5 = typedef "nirio_resource_hc.ctl" = tag
  T6 = typedef "user config.ctl" = cluster{"vst_device":refnum<k15>[], "RF gain ":dbl, "buffer size":u32, "center frequency (Hz) ":dbl, "P2P sample rate":dbl, "mode":enum16{"USRP - 180MHz", "5785 - 2*180MHz", "5785 - 3.2GHz", "P2P - VST"}, "devicess":T5[], "gen for df":bool, "Rx settings":cluster{"min PW         ":dbl, "max gap        ":dbl, "detection bar":dbl, "peak detect                        ":bool}, "use arb files":bool}
  T7 = typedef "PDW_lv2.ctl" = cluster{"t start":dbl, "frequency (Hz)":dbl, "duration (sec)":dbl, "mod type":T8, "mod depth":dbl, "trig":bool, "amp (lin)":dbl, "diraction (deg)":dbl, "phase(deg)":dbl}
  T8 = typedef "mode_type.ctl" = enum8{"CW", "from memory 1", "NC - cw", "LFM", "BPSK", "QPSK"}
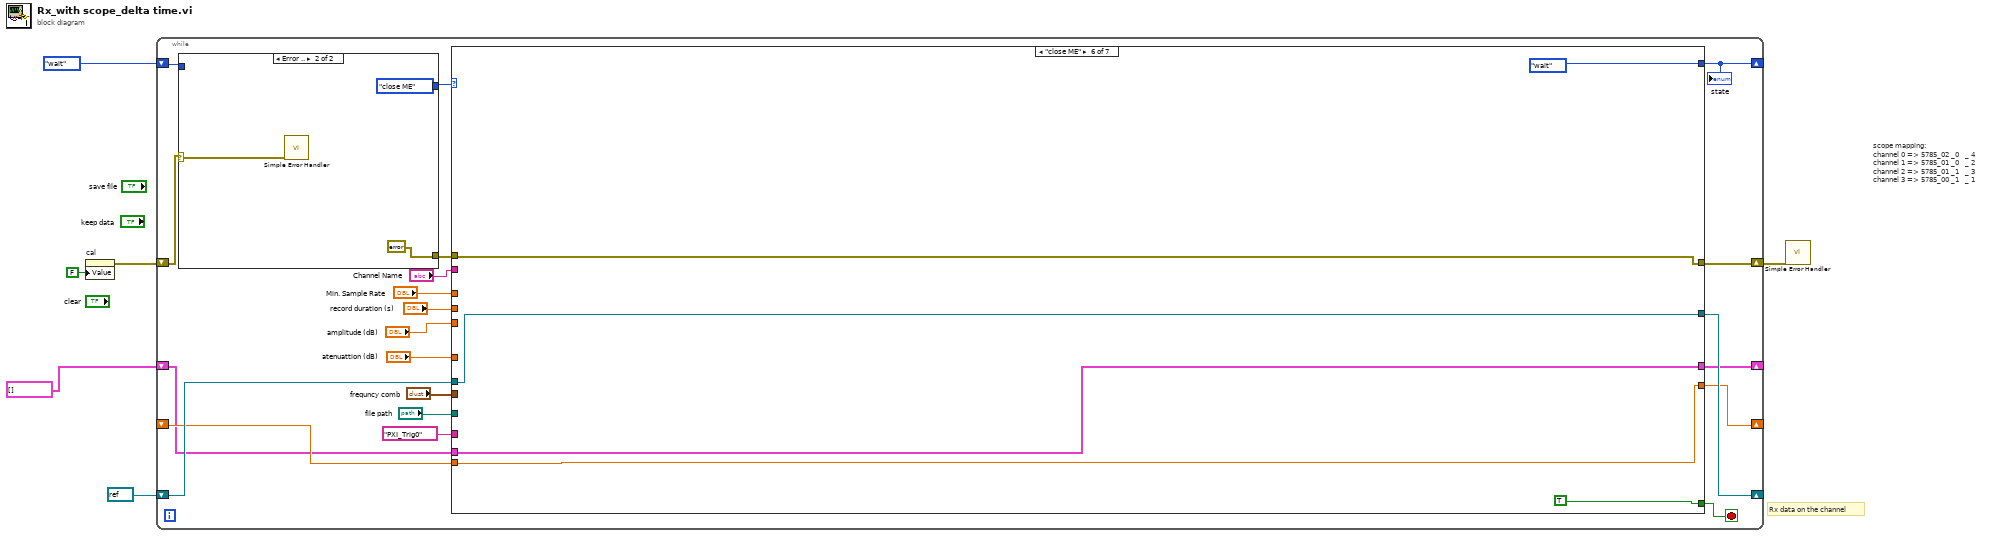
[diagram p0: block diagram]
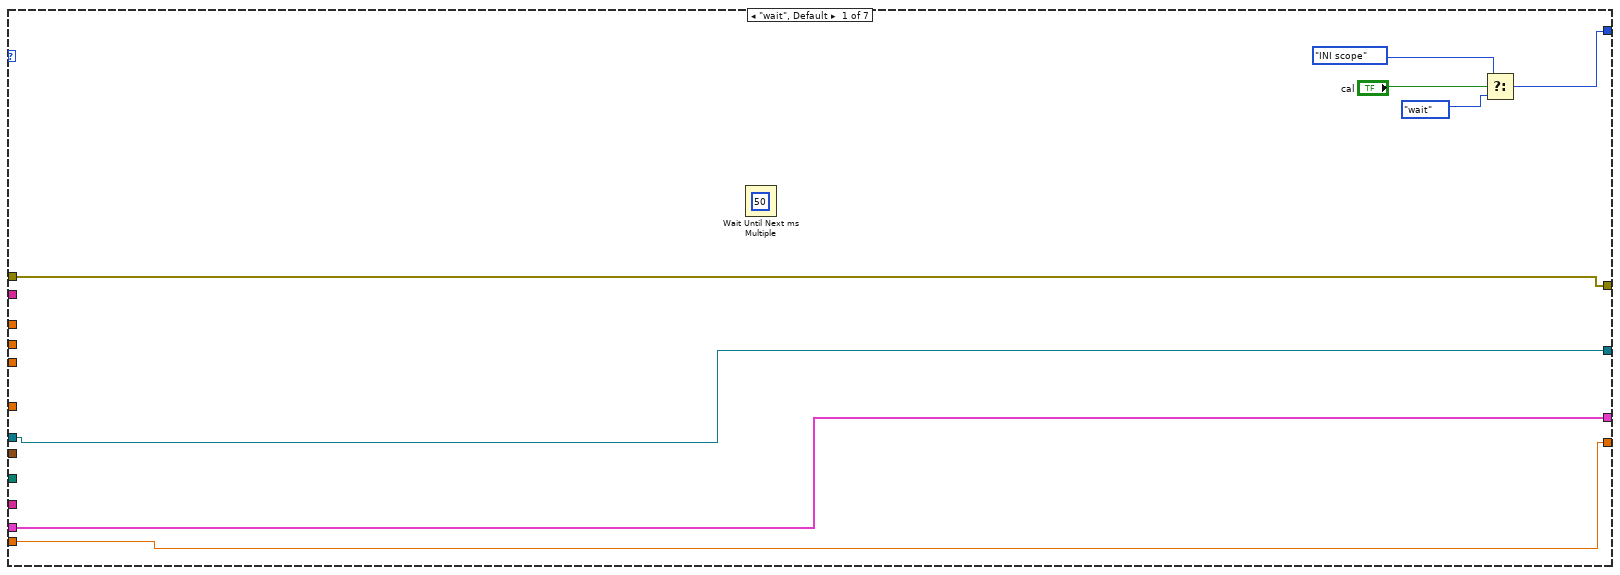
[diagram p2: hidden frame]
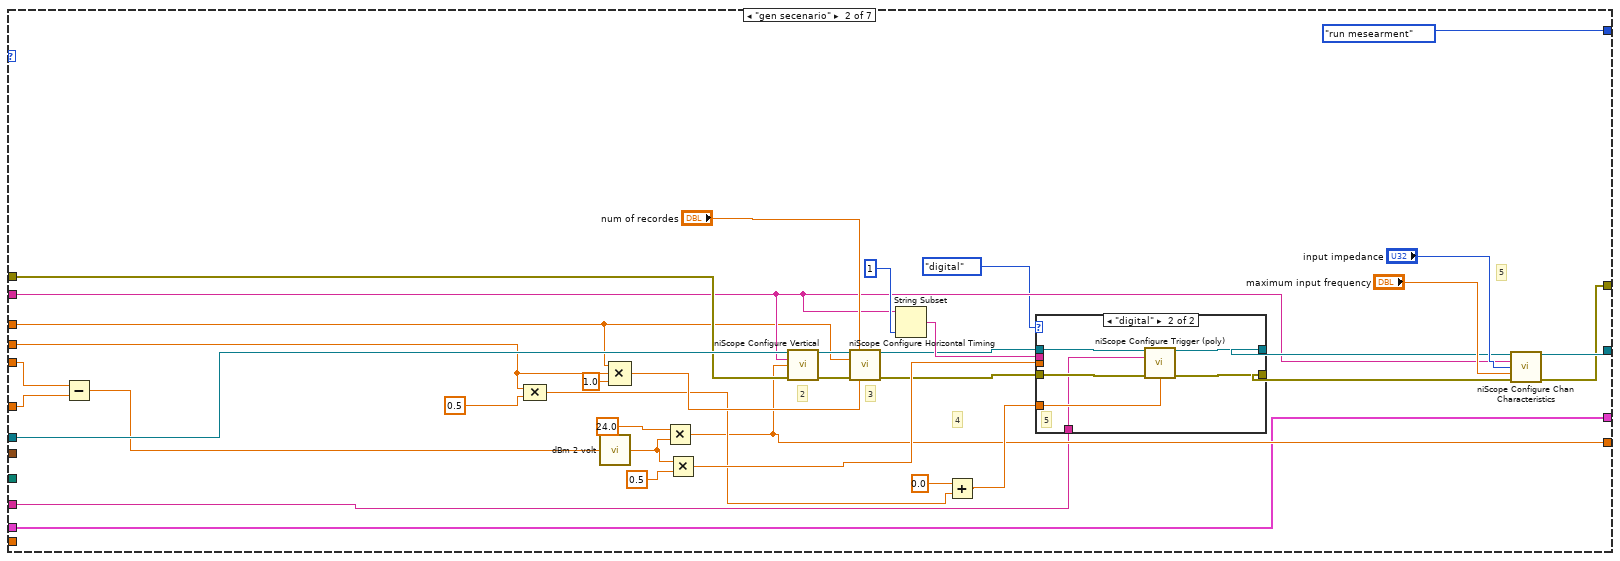
[diagram p3: hidden frame]
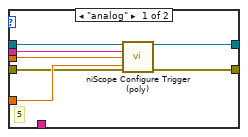
[diagram p4: hidden frame]
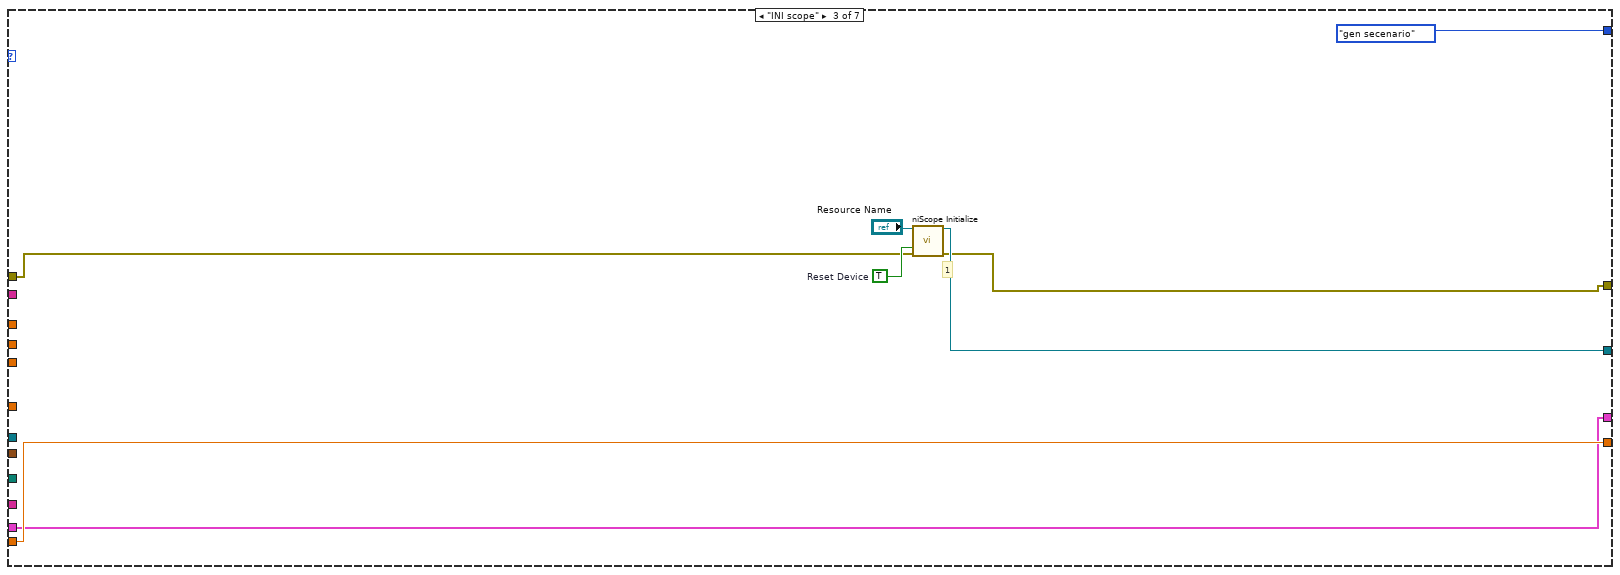
[diagram p5: hidden frame]
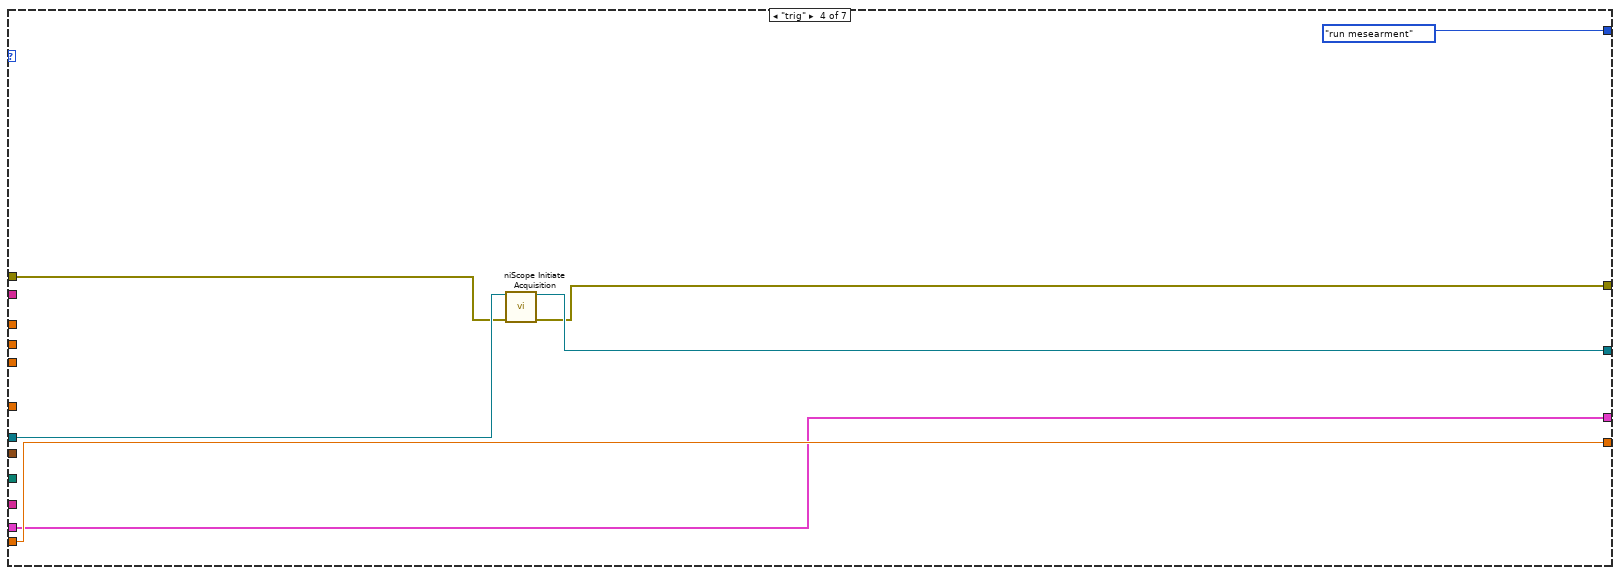
[diagram p6: hidden frame]
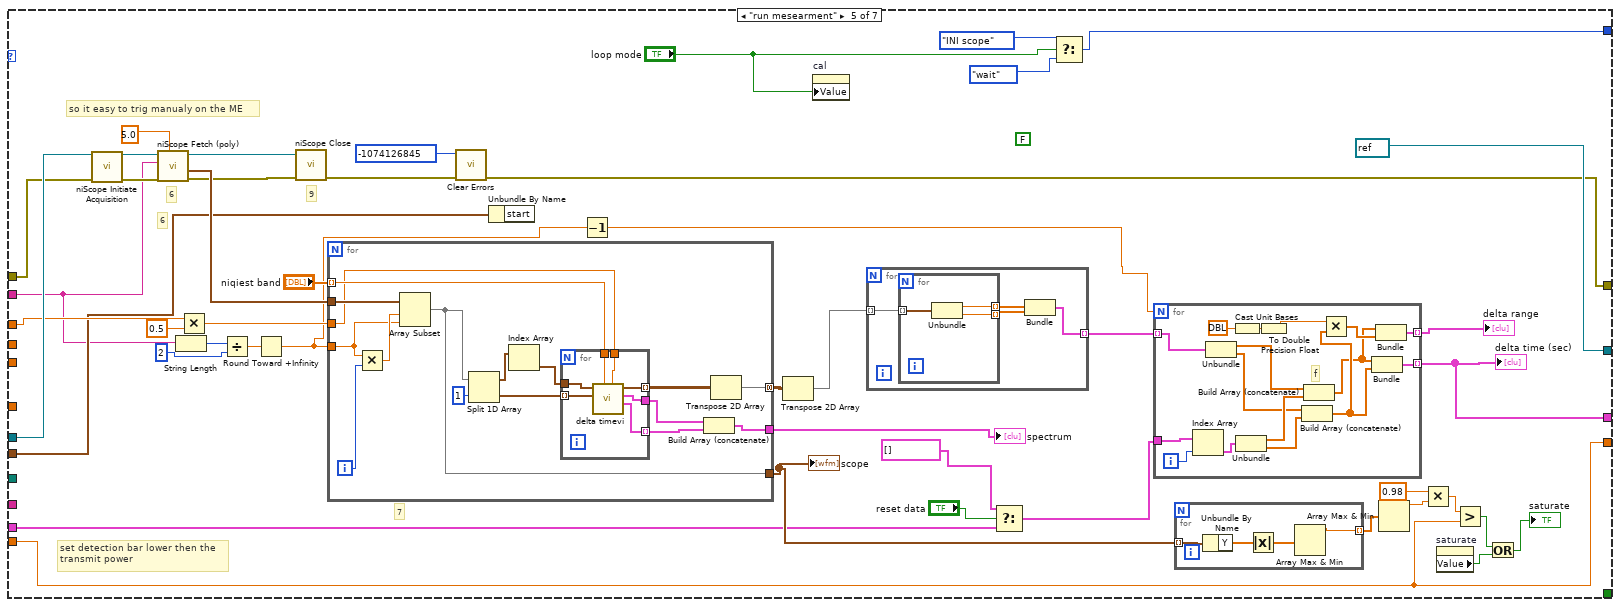
[diagram p7: hidden frame]
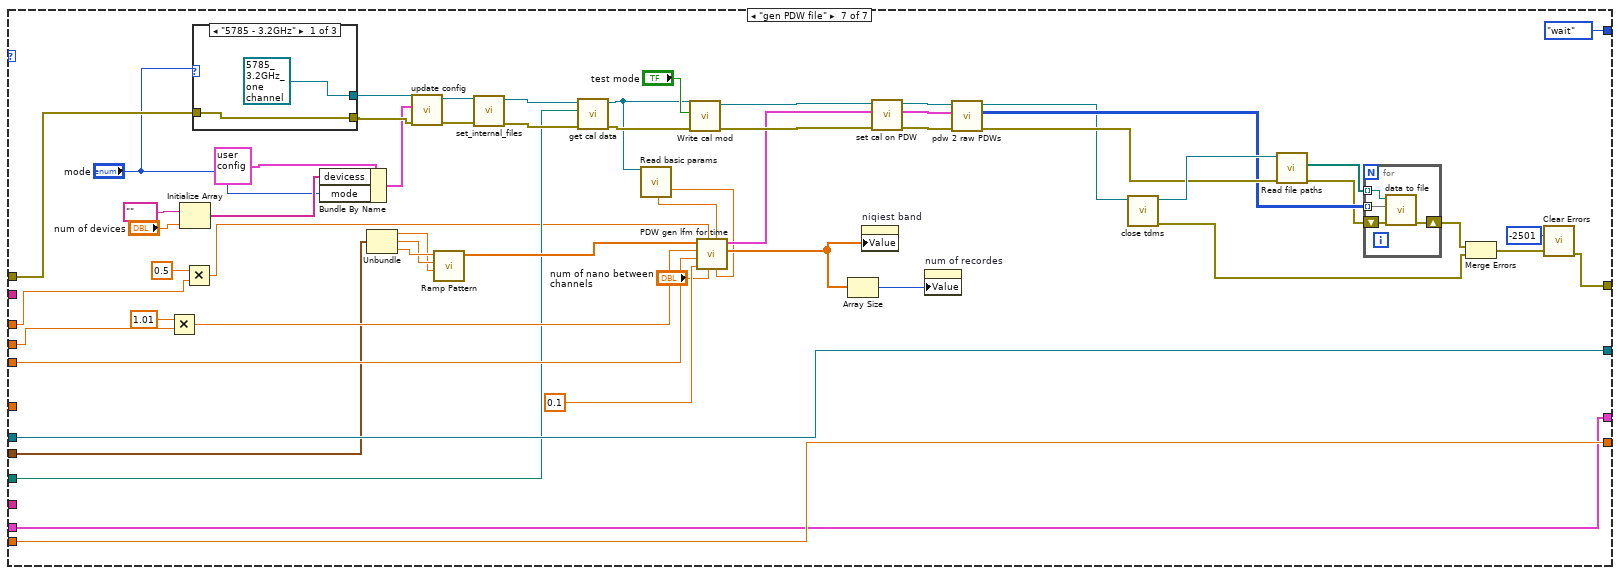
[diagram p8: hidden frame]
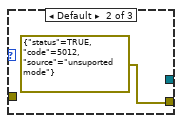
[diagram p9: hidden frame]
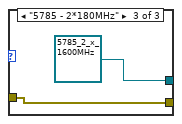
[diagram p10: hidden frame]
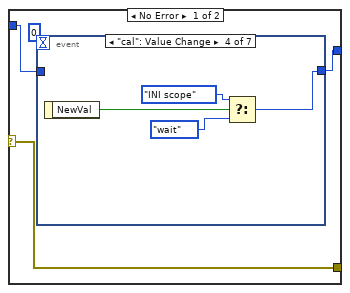
[diagram p11: hidden frame]
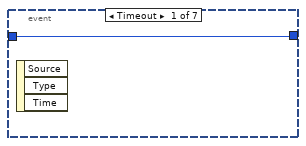
[diagram p12: hidden frame]
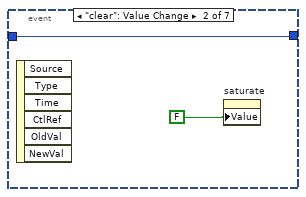
[diagram p13: hidden frame]
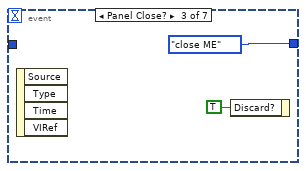
[diagram p14: hidden frame]
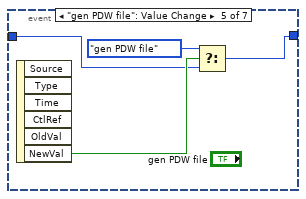
[diagram p15: hidden frame]
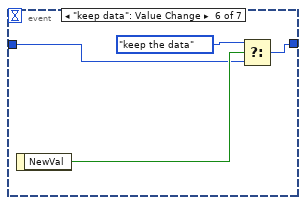
[diagram p16: hidden frame]
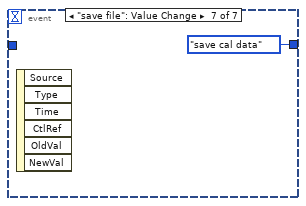
[diagram p17: hidden frame]
diagram:
  # "Rx data on the channel"
  # "scope mapping:\nchannel 0 => 5785_02 _0   _ 4\nchannel 1 => 5785_01 _0   _ 2 \nchannel 2 => 5785_01 _1   _ 3\nchannel 3 => 5785_00 _1   _ 1"
  n1 = property on="cal" class="Bool (strict)"("Value"=FALSE ("cal")) -> (error out=w2:errorcluster)  [unwired: 2 in, 1 out]
  n2 = while {
    shift-right: [w17] -> _
    shift-left: states_for_scope."wait" -> [w25]
    shift-right: [w23] -> w4
    shift-left: w2 -> [w27]
    shift-right: [w20] -> _
    shift-left: refnum<k15> refnum ("instrument handle out") -> [w19]
    shift-right: [w13] -> _
    shift-left: _ -> [w12]
    shift-right: [w8] -> _
    shift-left: cluster{dbl[], dbl[]}[] [] -> [w7]
    stop <- w16 stop-if-true
    n3 = case shown="Error .." w27 {
      selector: w27 -> [w271 w292]
      tunnel: [w269 states_for_scope."close ME"] -> w26
      tunnel: w25 -> [w270 _]
      tunnel: [w271 errorcluster {"status"=FALSE, "code"=0, "source"=""} ("error IO")] -> w24
      frame No Error {
        n4 = event shown="[3] \"cal\": Value Change" {
          selector: _ -> [_ _ _ _ _ _ _]
          dyn-events: _ -> [_ _ _ _ _ _ _]
          timeout: 0 -> [_ _ _ _ _ _ _]
          tunnel: w270 -> [w272 w274 _ _ w283 w286 _]
          tunnel: [w272 w274 states_for_scope."close ME" w278 w282 w285 states_for_scope."save cal data" ("f")] -> w269
          event Timeout {
            n5 = event-data() -> ()  [unwired: 1 in, 3 out]
          }
          event "clear": Value Change {
            n6 = event-data() -> ()  [unwired: 1 in, 6 out]
            n7 = property on="saturate" class="Bool (strict)"("Value"=FALSE ("clear")) -> ()  [unwired: 2 in, 2 out]
          }
          event Panel Close? {
            n8 = event-data() -> ()  [unwired: 1 in, 4 out]
            n9 = event-data("Discard?"=TRUE) -> ()  [unwired: 1 in, 1 out]
          }
          event "cal": Value Change {
            n10 = event-data() -> ("NewVal"=w280:bool)  [unwired: 1 in]
            n11 = Select(t=states_for_scope."INI scope", s=w280, f=states_for_scope."wait") -> (s? t:f=w278:T2)
          }
          event "gen PDW file": Value Change {
            n12 = event-data() -> ("NewVal"=w284:bool)  [unwired: 1 in, 5 out]
            n13 = Select(t=states_for_scope."gen PDW file", s=w284, f=w283) -> (s? t:f=w282:T2)
          }
          event "keep data": Value Change {
            n14 = event-data() -> ("NewVal"=w288:bool)  [unwired: 1 in]
            n15 = Select(t=states_for_scope."keep the data" ("f"), s=w288, f=w286) -> (s? t:f=w285:T2)
          }
          event "save file": Value Change {
            n16 = event-data() -> ()  [unwired: 1 in, 6 out]
          }
        }
      }
      frame Error {
        n17 = call <vilib>:"Simple Error Handler.vi"("error in (no error)"=w292) -> ()  [unwired: 4 in, 5 out]
      }
    }
    n18 = case shown="\"close ME\"" w26 {
      tunnel: w24 -> [w35 w57 w88 w97 w137 w199 w244]
      tunnel: [w35 w52 w90 w98 w133 w199 w248] -> w23
      tunnel: "record duration (s)" -> [_ w61 _ _ _ _ w238]
      tunnel: "amplitude (dB)" -> [_ w44 _ _ _ _ w235]
      tunnel: [w34 w53 w91 w99 refnum<k15> refnum ("instrument handle out") w200 w233] -> w20
      tunnel: w19 -> [w34 w62 _ w100 w139 w200 w233]
      tunnel: "Channel Name" -> [_ w49 _ _ w112 _ _]
      tunnel: [w30 states_for_scope."run mesearment" states_for_scope."gen secenario" states_for_scope."run mesearment" w140 states_for_scope."wait" states_for_scope."wait"] -> w17
      tunnel: [_ _ _ _ _ TRUE _] -> w16
      tunnel: "atenuattion (dB)" -> [_ w43 _ _ _ _ _]
      tunnel: "file path" -> [_ _ _ _ _ _ w217]
      tunnel: [w29 w41 w87 w95 w124 w198 w216] -> w13
      tunnel: w12 -> [w29 _ w87 w95 w124 w198 w216]
      tunnel: "Min. Sample Rate" -> [_ w40 _ _ w116 _ w214]
      tunnel: "frequncy comb" -> [_ _ _ _ w113 _ w210]
      tunnel: T3 "PXI_Trig0" ("trigger source") -> [_ w39 _ _ _ _ _]
      tunnel: [w28 w38 w86 w94 w103 w197 w206] -> w8
      tunnel: w7 -> [w28 w38 w86 w94 w102 w197 w206]
      frame "wait", Default {
        n19 = Wait Until Next ms Multiple(millisecond multiple=u32 50) -> ()  [unwired: 1 out]
        n20 = Select(t=states_for_scope."INI scope", s="cal", f=states_for_scope."wait") -> (s? t:f=w30:T2)
      }
      frame "gen secenario" {
        # "5"
        # "4"
        # "3"
        # "2"
        n21 = Subtract(x=w44, y=w43) -> (x-y=w42:dbl)
        n22 = Compound Arithmetic op=MULTIPLY(w61, 0.5 ("value")) -> (w47:dbl)
        n23 = call "dBm 2 volt.vi"("dBm"=w42) -> ("V"=w70:dbl)
        n24 = Compound Arithmetic op=MULTIPLY(w40, w61, 1.0 ("value")) -> (w72:dbl)
        n25 = Multiply(x=24.0, y=w70) -> (x*y=w41:dbl)
        n26 = Multiply(x=w70, y=0.5) -> (x*y=w71:dbl)
        n27 = call <instrlib>:"niScope Configure Vertical.vi"("instrument handle"=w62, "channels"=w49, "vertical range"=w41, "error in"=w57) -> ("instrument handle out"=w59:refnum<k15>, "error out"=w58:errorcluster)  [unwired: 10 in]
        n28 = call <instrlib>:"niScope Configure Horizontal Timing.vi"("instrument handle"=w59, "number of records"="num of recordes", "min sample rate"=w40, "error in"=w58, "min record length"=w72) -> ("instrument handle out"=w68:refnum<k15>, "error out"=w67:errorcluster)  [unwired: 9 in]
        n29 = String Subset(string=w49, length (rest)=1 ("length (rest)")) -> (substring=w69:string)  [unwired: 1 in]
        n30 = Add(x=0.0, y=w47) -> (x+y=w45:dbl)
        n31 = case shown="\"digital\"" scope_trig_type."digital" {
          tunnel: w71 -> [w79 _]
          tunnel: w45 -> [w78 w81]
          tunnel: w69 -> [w77 _]
          tunnel: w68 -> [w76 w85]
          tunnel: w67 -> [w75 w84]
          tunnel: [w74 w83] -> w54
          tunnel: [w73 w82] -> w51
          tunnel: w39 -> [_ w80]
          frame "analog" {
            # "5"
            n32 = call-poly <instrlib>:"niScope Configure Trigger (poly).vi"("instrument handle"=w76, "trigger source"=w77, "trigger level"=w79, "error in"=w75, "trigger delay"=w78) -> ("instrument handle out"=w74:refnum<k15>, "error out"=w73:errorcluster)  [unwired: 9 in]
          }
          frame "digital" {
            # "5"
            n33 = call-poly <instrlib>:"niScope Configure Trigger (poly).vi"("instrument handle"=w85, "trigger source"=w80, "error in"=w84, "trigger delay"=w81) -> ("instrument handle out"=w83:refnum<k15>, "error out"=w82:errorcluster)  [unwired: 10 in]
          }
        }
        n34 = call <instrlib>:"niScope Configure Chan Characteristics.vi"("instrument handle"=w54, "channels"=w49, "input impedance"="input impedance", "maximum input frequency"="maximum input frequency", "error in"=w51) -> ("instrument handle out"=w53:refnum<k15>, "error out"=w52:errorcluster)  [unwired: 9 in]
      }
      frame "INI scope" {
        w92 = TRUE  # Reset Device
        # "1"
        n35 = call <instrlib>:"niScope Initialize.vi"("resource name"="Resource Name", "reset device"=w92, "error in"=w88) -> ("instrument handle"=w91:refnum<k15>, "error out"=w90:errorcluster)  [unwired: 11 in]
      }
      frame "trig" {
        n36 = call <instrlib>:"niScope Initiate Acquisition.vi"("instrument handle"=w100, "error in"=w97) -> ("instrument handle out"=w99:refnum<k15>, "error out"=w98:errorcluster)  [unwired: 12 in]
      }
      frame "run mesearment" {
        (unwired) FALSE ("cal mode")
        # "so it easy to trig manualy on the ME"
        # "set detection bar lower then the\ntransmit power"
        # "6"
        # "9"
        # "7"
        # "6"
        n37 = call <instrlib>:"niScope Initiate Acquisition.vi"("instrument handle"=w139, "error in"=w137) -> ("instrument handle out"=w138:refnum<k15>, "error out"=w136:errorcluster)  [unwired: 12 in]
        n38 = call-poly <instrlib>:"niScope Fetch (poly).vi"("timeout"=5.0, "error in"=w136, "channels"=w112, "instrument handle"=w138) -> ("error out"=w144:errorcluster, "wfm"=w145:waveform(dbl)[], "instrument handle out"=w143:refnum<k15>)  [unwired: 4 in, 1 out]
        n39 = String Length(string=w112) -> (length=w110:i32)
        n40 = Multiply(x=w116, y=0.5) -> (x*y=w114:dbl)
        n41 = Divide(x=w110, y=2 ("x")) -> (x/y=w111:dbl)
        n42 = Round Toward +Infinity(x=w111) -> (ceil(x): smallest int >= x=w108:dbl)
        n43 = call <instrlib>:"niScope Close.vi"("instrument handle"=w143, "error in"=w144) -> ("error out"=w134:errorcluster)  [unwired: 13 in]
        n44 = for {
          tunnel: w145 -> [w189]
          tunnel: [w182] -> w146 mode=concatenating
          tunnel: [w181] -> w126
          tunnel: [w178] -> w128
          tunnel: "niqiest band" -> [w177] mode=indexing
          tunnel: w114 -> [w176]
          tunnel: w108 -> [w175]
          i -> [w188]
          n45 = Multiply(x=w175, y=w188) -> (x*y=w187:dbl)
          n46 = Array Subset(array=w189, index=w187, length=w175) -> (w181:waveform(dbl)[])
          n47 = Split 1D Array(array=w181, index=1) -> (first subarray=w174:waveform(dbl)[], second subarray=w184:waveform(dbl)[])
          n48 = Index Array(array=w174) -> (element=w185:waveform(dbl))  [unwired: 1 in]
          n49 = for {
            tunnel: w185 -> [w196]
            tunnel: w184 -> [w195] mode=indexing
            tunnel: [w190] -> w183 mode=indexing
            tunnel: [w194] -> w180
            tunnel: [w193] -> w179 mode=indexing
            tunnel: w177 -> [w192]
            tunnel: w176 -> [w191]
            n50 = call "delta timevi.vi"("niqiest frequecy"=w191, "niqiest band"=w192, "signal in 2"=w195, "signal in 1"=w196) -> ("PSD 1"=w193:cluster{"f0":dbl, "df":dbl, "magnitude":dbl[]}, "PSD 0"=w194:cluster{"f0":dbl, "df":dbl, "magnitude":dbl[]}, "d time"=w190:cluster{"frequncy":dbl, "d time":dbl}[])  [unwired: 5 in]
          }
          n51 = Build Array (concatenate)(w180, w179) -> (w178:cluster{"f0":dbl, "df":dbl, "magnitude":dbl[]}[])
          n52 = Transpose 2D Array(2D array=w183) -> (transposed array=w182:cluster{"frequncy":dbl, "d time":dbl}[][])
        }
        "scope" <- w126
        "spectrum" <- w128
        n53 = call <vilib>:"Clear Errors.vi"("error in (no error)"=w134, "specific error code to clear (0: all)"=-1074126845) -> ("error out"=w133:errorcluster)  [unwired: 4 in, 1 out]
        n54 = Unbundle By Name(w113) -> ()  [unwired: 1 out]
        n55 = Decrement(x=w108) -> (x-1=w107:dbl)
        n56 = Transpose 2D Array(2D array=w146) -> (transposed array=w106:cluster{"frequncy":dbl, "d time":dbl}[][])
        n57 = property on="cal" class="Bool (strict)"("Value"="loop mode") -> ()  [unwired: 2 in, 2 out]
        n58 = for {
          tunnel: w106 -> [w150] mode=indexing
          tunnel: [w147] -> w105 mode=indexing
          n59 = for {
            tunnel: w150 -> [w153] mode=indexing
            tunnel: [w152] -> w149 mode=indexing
            tunnel: [w151] -> w148 mode=indexing
            n60 = Unbundle(w153) -> ("frequncy"=w152:dbl, "d time"=w151:dbl)
          }
          n61 = Bundle(w149, w148) -> (w147:cluster{dbl[], dbl[]})  [unwired: 1 in]
        }
        n62 = Select(t=cluster{dbl[], dbl[]}[] [], s="reset data", f=w102) -> (s? t:f=w130:cluster{dbl[], dbl[]}[])
        n63 = Select(t=states_for_scope."INI scope", s="loop mode", f=states_for_scope."wait") -> (s? t:f=w140:T2)
        n64 = for {
          N: w107 -> [_]
          tunnel: w130 -> [w173]
          tunnel: [w169] -> w103 mode=indexing
          tunnel: w105 -> [w167] mode=indexing
          tunnel: [w158] -> w101 mode=indexing
          i -> [w168]
          # "f"
          n65 = Index Array(array=w173, index=w168) -> (element=w172:cluster{dbl[], dbl[]})
          n66 = Unbundle(w167) -> (w165:dbl[], w162:dbl[])
          n67 = Cast Unit Bases(0:ext[unit] 299792458.0) -> (2:w166:ext)  [unwired: 1 in]
          n68 = Unbundle(w172) -> (w171:dbl[], w170:dbl[])
          n69 = To Double Precision Float(number=w166) -> (double precision float=w163:dbl)
          n70 = Build Array (concatenate)(w162, w170) -> (w161:dbl[])
          n71 = Build Array (concatenate)(w165, w171) -> (w159:dbl[])
          n72 = Multiply(x=w163, y=w161) -> (x*y=w160:dbl[])
          n73 = Bundle(w159, w161) -> (w169:cluster{dbl[], dbl[]})  [unwired: 1 in]
          n74 = Bundle(w159, w160) -> (w158:cluster{dbl[], dbl[]})  [unwired: 1 in]
        }
        "delta time (sec)" <- w103
        "delta range" <- w101
        n75 = for {
          tunnel: w126 -> [w157] mode=indexing
          tunnel: [w156] -> w125 mode=indexing
          n76 = Unbundle By Name(w157) -> ("Y"=w155:dbl[])
          n77 = Absolute Value(x=w155) -> (abs(x)=w154:dbl[])
          n78 = Array Max & Min(array=w154) -> (max value=w156:dbl)  [unwired: 3 out]
        }
        n79 = Array Max & Min(array=w125) -> (max value=w123:dbl)  [unwired: 3 out]
        n80 = Multiply(x=0.98, y=w123) -> (x*y=w121:dbl)
        n81 = property on="saturate" class="Bool (strict)"() -> ("Value"=w120:bool)  [unwired: 2 in, 2 out]
        n82 = Greater?(x=w121, y=w124) -> (0:w119:bool)
        n83 = Or(x=w119, y=w120) -> (x .or. y?=→"saturate":bool)
      }
      frame "close ME" {
      }
      frame "gen PDW file" {
        n84 = Multiply(x=1.01, y=w238) -> (x*y=w236:dbl)
        n85 = Initialize Array(T5 "" ("resource name"), "num of devices") -> (w229:T5[])
        n86 = Multiply(x=0.5, y=w214) -> (x*y=w213:dbl)
        n87 = case shown="\"5785 - 3.2GHz\"" "mode" {
          tunnel: [refnum<class "5785_3.2GHz_one channel.lvclass"> refnum ("5785_3.2GHz_one channel.lvclass") _ refnum<class "5785_2_x_1600MHz.lvclass"> refnum ("5785_2_x_1600MHz.lvclass")] -> w245
          tunnel: w244 -> [w259 _ w262]
          tunnel: [w259 errorcluster {"status"=TRUE, "code"=5012, "source"="unsuported mode"} ("error IO") w262] -> w243
          frame "5785 - 3.2GHz" {
          }
          frame Default {
          }
          frame "5785 - 2*180MHz" {
          }
        }
        n88 = Bundle By Name(cluster=T6 {"vst_device"=["VST_1", "VST_2"], "RF gain "=10.0, "buffer size"=524288, "center frequency (Hz) "=1000000000.0, "P2P sample rate"=200000000.0, "mode"=enum."5785 - 2*180MHz", "devicess"=["IF_transiver_0", "IF_transiver_1", "IF_transiver_2"], "gen for df"=TRUE, "Rx settings"={"min PW         "=0.0, "max gap        "=0.0, "detection bar"=0.0, "peak detect                        "=FALSE}, "use arb files"=FALSE} ("user configurations"), "devicess"=w229, "mode"="mode") -> (w228:T6)
        n89 = Unbundle(w210) -> ("start"=w240:dbl, "end"=w241:dbl, "delta"=w242:dbl)
        n90 = call-dynamic "update config.vi"("error in (no error)"=w243, "user configurations"=w228, "device_type in"=w245) -> ("error out"=w246:errorcluster, "device_type out"=w247:refnum<class "device_type.lvclass">)  [unwired: 5 in, 2 out]
        n91 = call-poly <vilib>:"Ramp Pattern.vi"("start"=w240, "end"=w241, "delta"=w242) -> ("Ramp Pattern"=w239:dbl[])  [unwired: 6 in, 2 out]
        n92 = call-dynamic "set_internal_files.vi"("error in (no error)"=w246, "device_type in"=w247) -> ("error out"=w219:errorcluster, "device_type out"=w220:refnum<class "device_type.lvclass">)  [unwired: 8 in]
        n93 = call-dynamic "get cal data.vi"("error in (no error)"=w219, "cal file path"=w217, "device_type in"=w220) -> ("error out"=w218:errorcluster, "device_type out"=w208:refnum<class "device_type.lvclass">)  [unwired: 7 in]
        n94 = call-dynamic "Read basic params.vi"("device_type in"=w208) -> ("number of channels"=w207:dbl, "center frequency (Hz)"=w203:dbl)  [unwired: 11 in, 6 out]
        n95 = call-dynamic "Write cal mod.vi"("error in (no error)"=w218, "apply cal data"="test mode", "device_type in"=w208) -> ("error out"=w224:errorcluster, "device_type out"=w225:refnum<class "device_type.lvclass">)  [unwired: 7 in]
        n96 = call "PDW gen lfm for time.vi"("center freqency"=w203, "num of channels"=w207, "num of nano between channels"="num of nano between channels", "niqiest freqency"=w213, "D.C"=0.1, "pulse amplitude"=w235, "pulse duration"=w236, "frequency list"=w239) -> ("niqiest band"=w211:dbl[], "PDWs on channels"=w209:cluster{T7[]}[])  [unwired: 2 in]
        n97 = Array Size(array=w211) -> (size(s)=w212:i32)
        n98 = property on="niqiest band" class="Arr (strict)"("Value"=w211) -> ()  [unwired: 2 in, 2 out]
        n99 = call "set cal on PDW.vi"("error in (no error)"=w224, "PDWs on channels"=w209, "device_type in"=w225) -> ("error out"=w223:errorcluster, "PDWs on channels"=w222:cluster{T7[]}[], "device_type out"=w221:refnum<class "device_type.lvclass">)  [unwired: 6 in]
        n100 = property on="num of recordes" class="DigNum (strict)"("Value"=w212) -> ()  [unwired: 2 in, 2 out]
        n101 = call-dynamic "pdw 2 raw PDWs.vi"("error in (no error)"=w223, "PDWs on channels"=w222, "device_type in"=w221) -> ("error out"=w254:errorcluster, "Array"=w252:u64[][], "device_type out"=w227:refnum<class "device_type.lvclass">)  [unwired: 6 in]
        n102 = call-dynamic "close tdms.vi"("device_type in"=w227) -> ("error out"=w257:errorcluster, "device_type out"=w255:refnum<class "device_type.lvclass">)  [unwired: 9 in]
        n103 = call-dynamic "Read file paths.vi"("error in (no error)"=w254, "device_type in"=w255) -> ("error out"=w251:errorcluster, "file paths"=w253:path[])  [unwired: 6 in, 2 out]
        n104 = for {
          tunnel: w252 -> [w265] mode=indexing
          shift-right: [w266] -> w256
          shift-left: w251 -> [w267]
          tunnel: w253 -> [w264] mode=indexing
          n105 = call "data to file.vi"("error in (no error)"=w267, "Array"=w265, "Path"=w264) -> ("error out"=w266:errorcluster)  [unwired: 8 in]
        }
        n106 = Merge Errors(w256, w257) -> (w258:errorcluster)
        n107 = call <vilib>:"Clear Errors.vi"("error in (no error)"=w258, "specific error code to clear (0: all)"=-2501) -> ("error out"=w248:errorcluster)  [unwired: 4 in, 1 out]
      }
    }
    "state" <- w17
  }
  n108 = call <vilib>:"Simple Error Handler.vi"("error in (no error)"=w4) -> ()  [unwired: 4 in, 5 out]
